vi "TOML-to-tree-recursive.vi"(5 "tag":string, 7 "name":string, 10 "value":T1, 11 "tree-control-ref":refnum<vi>) -> (0 "error out":errorcluster)   [LabVIEW 2020, in "TOML.lvlib"]
uses:
  TOML.lvlib
  TOML Value.ctl
  TOML Key-Value Pair.ctl
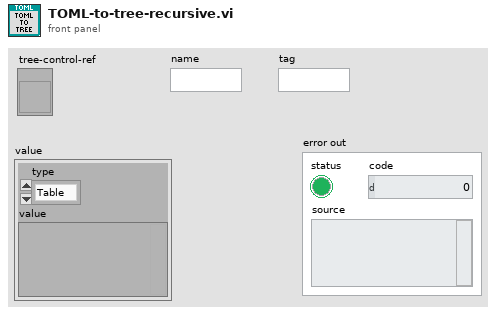
[diagram p1: front panel]
types:
  T1 = typedef "TOML.lvlib/TOML Value.ctl" = cluster{"type":enum16{"Table", "Array", "String", "Integer", "Float", "Boolean", "Offset Date-Time", "Local Date-Time", "Local Date", "Local Time", "Path"}, "value":variant}
  T2 = enum16{"Table", "Array", "String", "Integer", "Float", "Boolean", "Offset Date-Time", "Local Date-Time", "Local Date", "Local Time", "Path"}
  T3 = typedef "TOML.lvlib/TOML Key-Value Pair.ctl" = cluster{"Key":string, "Value":T1}
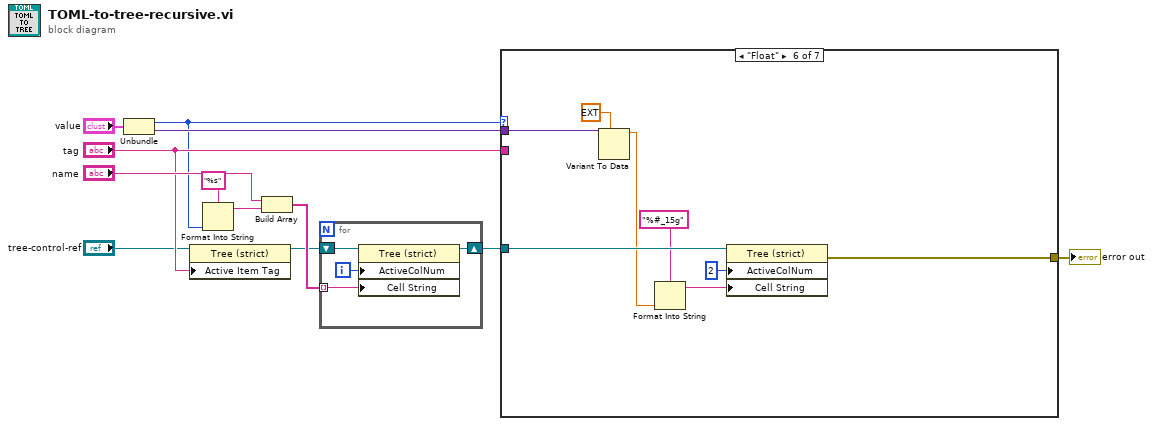
[diagram p0: block diagram]
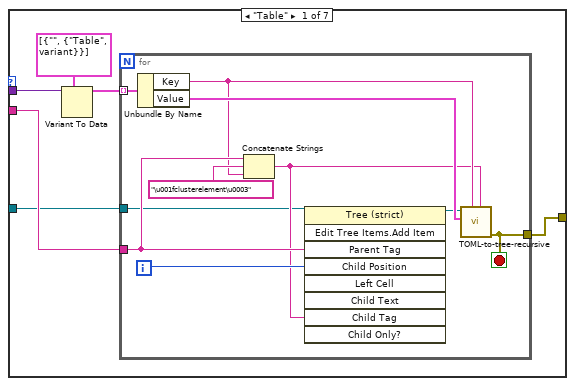
[diagram p2: hidden frame]
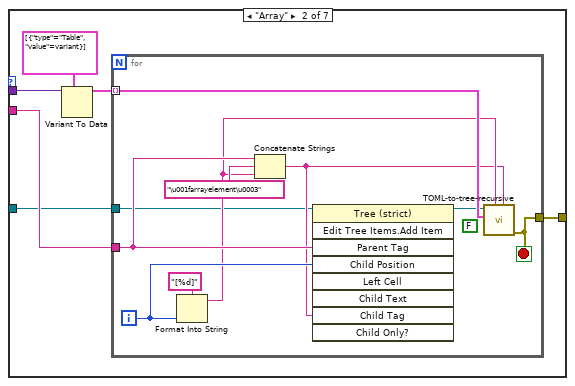
[diagram p3: hidden frame]
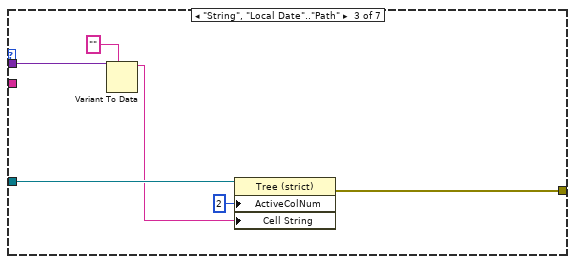
[diagram p4: hidden frame]
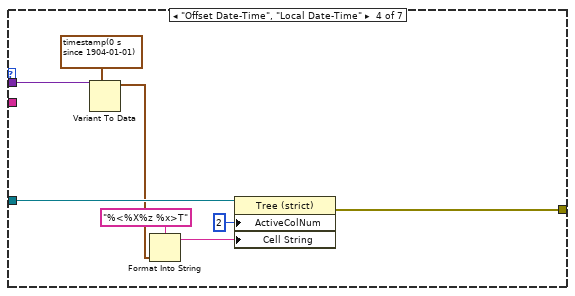
[diagram p5: hidden frame]
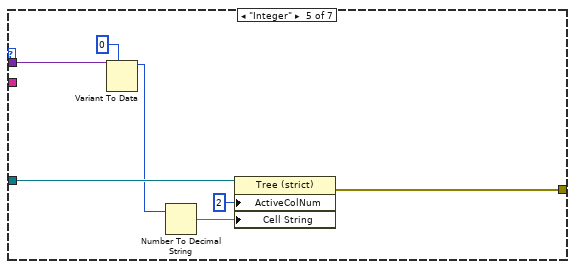
[diagram p6: hidden frame]
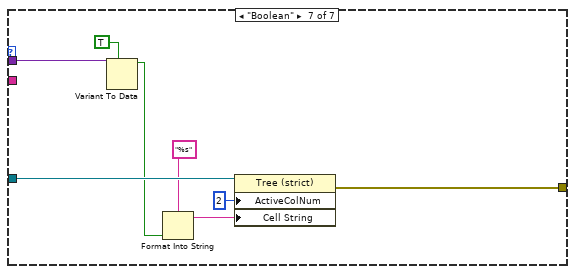
[diagram p7: hidden frame]
diagram:
  n1 = Unbundle("value") -> ("type"=w7:T2, "value"=w9:variant)
  n2 = property class="Tree (strict)"(reference="tree-control-ref", "Active Item Tag"="tag") -> (reference out=w4:refnum<vi>)  [unwired: 1 in, 1 out]
  n3 = Format Into String(format string="%s", w7) -> (resulting string=w6:string)  [unwired: 2 in, 1 out]
  n4 = Build Array("name", w6) -> (w5:string[])
  n5 = for {
    tunnel: w5 -> [w15] mode=indexing
    shift-right: [w13] -> w2
    shift-left: w4 -> [w16]
    i -> [w14]
    n6 = property class="Tree (strict)"(reference=w16, "ActiveColNum"=w14, "Cell String"=w15) -> (reference out=w13:refnum<vi>)  [unwired: 1 in, 1 out]
  }
  n7 = case shown="\"Float\"" w7 {
    tunnel: w9 -> [w22 w38 w54 w62 w69 w77 w85]
    tunnel: w2 -> [w18 w34 w52 w61 w68 w76 w84]
    tunnel: "tag" -> [w19 w35 _ _ _ _ _]
    tunnel: [w17 w33 w49 w55 w63 w70 w78] -> w1
    frame "Table" {
      n8 = Variant To Data(type=T3[] [{"Key"="", "Value"={"type"=enum."Table", "value"=variant}}], Variant=w22) -> (data=w20:T3[])  [unwired: 1 in, 1 out]
      n9 = for {
        tunnel: w20 -> [w32] mode=indexing
        tunnel: w19 -> [w29]
        tunnel: w18 -> [w24]
        tunnel: [w23] -> w17
        i -> [w28]
        stop <- w23 stop-if-true
        n10 = Unbundle By Name(w32) -> ("Key"=w27:string, "Value"=w31:T1)
        n11 = Concatenate Strings(w29, "\u001fclusterelement\u0003" ("string"), w27) -> (w26:string)
        n12 = invoke class="Tree (strict)" method="Edit Tree Items.Add Item"(reference=w24, "Parent Tag"=w29, "Child Position"=w28, "Child Tag"=w26) -> (reference out=w25:refnum<vi>)  [unwired: 5 in, 8 out]
        n13 = call "TOML-to-tree-recursive.vi"("tag"=w26, "name"=w27, "value"=w31, "tree-control-ref"=w25) -> ("error out"=w23:errorcluster)  [unwired: 7 in]
      }
    }
    frame "Array" {
      n14 = Variant To Data(type=T1[] [{"type"=enum."Table", "value"=variant}], Variant=w38) -> (data=w36:T1[])  [unwired: 1 in, 1 out]
      n15 = for {
        tunnel: w36 -> [w46] mode=indexing
        tunnel: w35 -> [w47]
        tunnel: w34 -> [w40]
        tunnel: [w39] -> w33
        i -> [w45]
        stop <- w39 stop-if-true
        (unwired) FALSE ("purge")
        n16 = Format Into String(format string="[%d]", w45) -> (resulting string=w43:string)  [unwired: 2 in, 1 out]
        n17 = Concatenate Strings(w47, "\u001farrayelement\u0003" ("string"), w43) -> (w42:string)
        n18 = invoke class="Tree (strict)" method="Edit Tree Items.Add Item"(reference=w40, "Parent Tag"=w47, "Child Position"=w45, "Child Tag"=w42) -> (reference out=w41:refnum<vi>)  [unwired: 5 in, 8 out]
        n19 = call "TOML-to-tree-recursive.vi"("tag"=w42, "name"=w43, "value"=w46, "tree-control-ref"=w41) -> ("error out"=w39:errorcluster)  [unwired: 7 in]
      }
    }
    frame "String", "Local Date".."Path" {
      n20 = Variant To Data(type="", Variant=w54) -> (data=w50:string)  [unwired: 1 in, 1 out]
      n21 = property class="Tree (strict)"(reference=w52, "ActiveColNum"=2 ("Active Cell:Active Column Number"), "Cell String"=w50) -> (error out=w49:errorcluster)  [unwired: 1 in, 1 out]
    }
    frame "Offset Date-Time", "Local Date-Time" {
      n22 = Variant To Data(type=timestamp(0 s since 1904-01-01), Variant=w62) -> (data=w58:timestamp)  [unwired: 1 in, 1 out]
      n23 = Format Into String(format string="%<%X%z %x>T", w58) -> (resulting string=w57:string)  [unwired: 2 in, 1 out]
      n24 = property class="Tree (strict)"(reference=w61, "ActiveColNum"=2 ("Active Cell:Active Column Number"), "Cell String"=w57) -> (error out=w55:errorcluster)  [unwired: 1 in, 1 out]
    }
    frame "Integer" {
      n25 = Variant To Data(type=i64 0, Variant=w69) -> (data=w66:i64)  [unwired: 1 in, 1 out]
      n26 = Number To Decimal String(number=w66) -> (decimal integer string=w64:string)  [unwired: 1 in]
      n27 = property class="Tree (strict)"(reference=w68, "ActiveColNum"=2 ("Active Cell:Active Column Number"), "Cell String"=w64) -> (error out=w63:errorcluster)  [unwired: 1 in, 1 out]
    }
    frame "Float" {
      n28 = Variant To Data(type=ext 0.0, Variant=w77) -> (data=w73:ext)  [unwired: 1 in, 1 out]
      n29 = Format Into String(format string="%#_15g", w73) -> (resulting string=w72:string)  [unwired: 2 in, 1 out]
      n30 = property class="Tree (strict)"(reference=w76, "ActiveColNum"=2 ("Active Cell:Active Column Number"), "Cell String"=w72) -> (error out=w70:errorcluster)  [unwired: 1 in, 1 out]
    }
    frame "Boolean" {
      n31 = Variant To Data(type=TRUE, Variant=w85) -> (data=w81:bool)  [unwired: 1 in, 1 out]
      n32 = Format Into String(format string="%s", w81) -> (resulting string=w80:string)  [unwired: 2 in, 1 out]
      n33 = property class="Tree (strict)"(reference=w84, "ActiveColNum"=2 ("Active Cell:Active Column Number"), "Cell String"=w80) -> (error out=w78:errorcluster)  [unwired: 1 in, 1 out]
    }
  }
  "error out" <- w1
